vi "Get Time Settings.vi"() -> (3 "DateTime":T1)   [LabVIEW 2015, in "SMI.lvlib"]
uses:
  SMI.lvlib
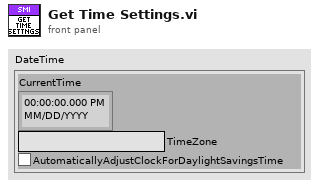
[diagram p1: front panel]
types:
  T1 = cluster{"CurrentTime":timestamp, "TimeZone":string, "AutomaticallyAdjustClockForDaylightSavingsTime":bool}
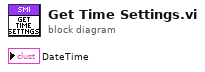
[diagram p0: block diagram]
diagram:
